vi "_PC_Err get_errcode_message.vi"(0 "err code":i32=11000, 1 "sourceError":string) -> (2 "err msg":string, 3 "customError":bool)   [LabVIEW 2018]
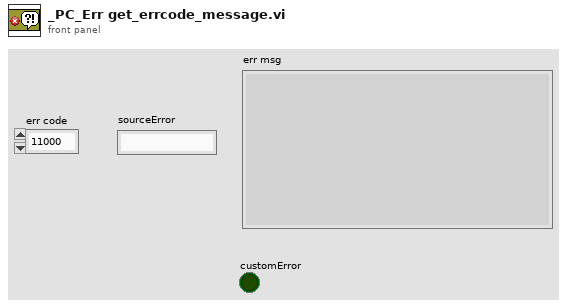
[diagram p1: front panel]
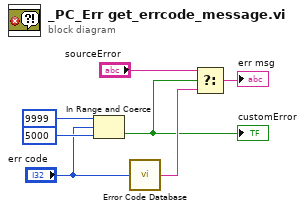
[diagram p0: block diagram]
diagram:
  n1 = In Range and Coerce(upper limit=9999 ("code"), x="err code", lower limit=5000 ("code")) -> (In Range?=w3:bool)  [unwired: 1 out]
  "customError" <- w3
  n2 = call <vilib>:"Error Code Database.vi"("Error Code"="err code") -> ("Error Text"=w7:string)
  n3 = Select(t="sourceError", s=w3, f=w7) -> (s? t:f=→"err msg":string)
